vi "Multichannel Recording0.9E.vi"() -> ()   [LabVIEW 2014]
uses:
  MultiChannelScheduling 1/Enum State Typedef.ctl
  MultiChannelScheduling 1/Consumer Data_ Consumer Event Com.ctl
  MultiChannelScheduling 1/Data Producer States.ctl
  <vilib>/_DAQmxBase/Internals/DAQmxBase Read (Analog 2D DBL NChan NSamp).vi
  <vilib>/_DAQmxBase/Internals/DAQmxBase Create Channel (AI-Voltage-Basic).vi
  <vilib>/_DAQmxBase/Internals/DAQmxBase Timing (Sample Clock).vi
panel:
  out "Recording Progress (% )":dbl(slide) scale=0.0..1.0
  in  "Display Size":T1(ring)
  out "Total Iterations Needed":dbl
  out "Read Data":i32
  out "Data Producer State":T2=enum."Default"
  out "Data Consumer State":T3=enum."Default"
  in  "Open Button":bool
  in  "Tab Control":T4(tab)
  in  "Amplifier Channel 0":T5 {"Amplifier Model" items=["Select a Model", "AM 1700", "BMA 200"]}
  out "Channel 0 Graph":waveform(dbl)(graph)
  in  "User Data Channel 0":T6
  in  "Use Channel 0":bool caption="In Use?"
  out "Channel 1 Graph":waveform(dbl)(graph)
  in  "User Data Channel 1":T6
  in  "Amplifier Channel 1":T5 {"Amplifier Model" items=["Select a Model", "AM 1700", "BMA 200"]}
  in  "Use Channel 1":bool caption="In Use?"
  out "Channel 2 Graph":waveform(dbl)(graph)
  in  "User Data Channel 2":T6
  in  "Amplifier Channel 2":T5 {"Amplifier Model" items=["Select a Model", "AM 1700", "BMA 200"]}
  in  "Use Channel 2":bool caption="In Use?"
  out "Channel 3 Graph":waveform(dbl)(graph)
  in  "User Data Channel 3":T6
  in  "Amplifier Channel 3":T5 {"Amplifier Model" items=["Select a Model", "AM 1700", "BMA 200"]}
  in  "Use Channel 3":bool caption="In Use?"
  out "Overview Graph":waveform(dbl)[](graph)
  in  "Stop Preview":bool
  in  "OK Button":bool
  out "Event State":T7
  in  "Clear Display":bool
  in  "Preview Button":bool
  out "Iterations Recorded":i32
  in  "Recording Time (s)":dbl
  in  "Sample Rate":i64=1000
  in  "Stop Button":bool
  out "Start Time hr/min":string
  out "Date mm/dd/yy":string
  in  "Exit Button":bool
  in  "Record Button":bool
  # "MSU EFISH Lab Multi-Channel Electronic Pulse Recorder v0.9E (Beta 6)"
  # "Setup"
  # "Must set sample rate before you press start"
  # "Preview"
  # "Recording"
  # "Blue for On\nOrange for Off"
  # "DC"
  # "AC"
  # "Blue for AC and Orange for DC"
  # "Blue for On\nOrange for Off"
  # "DC"
  # "AC"
  # "Blue for AC and Orange for DC"
  # "Blue for On\nOrange for Off"
  # "DC"
  # "AC"
  # "Blue for AC and Orange for DC"
  # "Blue for On\nOrange for Off"
  # "DC"
  # "AC"
  # "Blue for AC and Orange for DC"
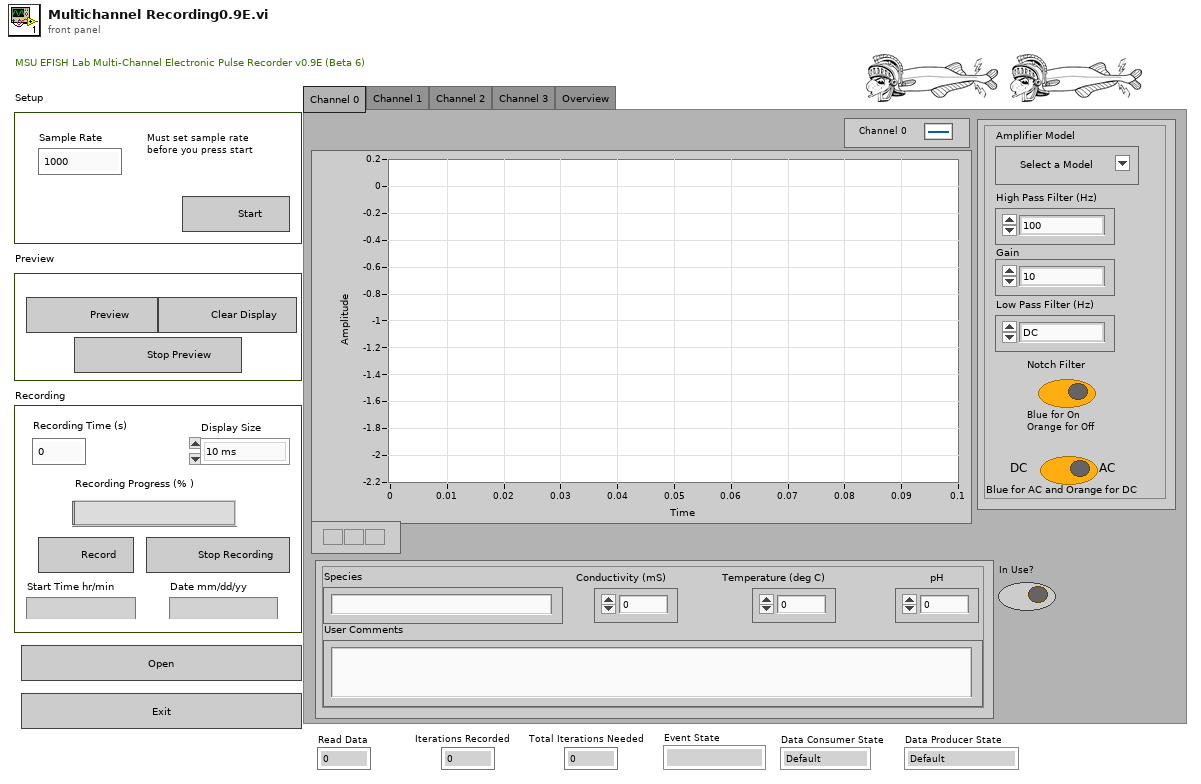
[diagram p1: front panel]
types:
  T1 = enum16{"10 ms", "100 ms", "1 Second", "10 sec", "30 sec"}
  T2 = typedef "Data Producer States.ctl" = enum16{"Read Data", "Set Sample Clock", "Default", "Exit", "Preview"}
  T3 = typedef "Consumer Data_ Consumer Event Com.ctl" = enum16{"Recording", "Create File", "Clear Memory", "Default", "End File", "Exit", "Set Sample Clock", "Preview"}
  T4 = enum32{"Channel 0", "Channel 1", "Channel 2", "Channel 3", "Overview"}
  T5 = cluster{"Low Pass Filter (Hz)":enum16{"DC", "0.1", "1", "3", "10", "30", "100", "300"}, "Gain ":enum16{"10", "20", "50", "100", "200", "500", "1000", "2k", "5k", "10k", "20k", "50k"}, "High Pass Filter (Hz)":enum16{"100", "500", "1000", "3000", "5000", "10,000", "20,000", "30,000", "50,000"}, "Notch Filter":bool, "Amplifier Model":u16, "AC/DC Switch":bool}
  T6 = cluster{"pH":dbl, "Conductivity (mS)":dbl, "Temperature (deg C)":dbl, "User Comments":string, "Species":string}
  T7 = typedef "Enum State Typedef.ctl" = enum16{"", "Open FIle", "Beginning State", "Set the Sample Clock", "Prepreview Handling", "Clear Display", "Preview Data", "Stop", "Exit", "Record", "Create File"}
  T8 = enum8{"Enabled", "Disabled", "Disabled and Grayed Out"}
  T9 = enum16{"Recording", "Create File", "Clear Memory", "Default"}
  T10 = cluster{"Refnum out":refnum<k34>, "Refnum out":refnum<k34>, "Refnum out":refnum<k34>, "Refnum out":refnum<k34>}
  T11 = cluster{"Use Channel 0":bool, "Use Channel 1":bool, "Use Channel 2":bool, "Use Channel 3":bool}
  T12 = cluster{"tdms file out":refnum<k34>, "tdms file out":refnum<k34>, "tdms file out":refnum<k34>, "tdms file out":refnum<k34>}
  T13 = cluster{"Waveform":waveform(dbl), "Waveform":waveform(dbl), "Waveform":waveform(dbl), "Waveform":waveform(dbl), waveform(dbl)[]}
  T14 = cluster{"Channel 0 Graph":refnum<vi>, "Channel 1 Graph":refnum<vi>, "Channel 2 Graph":refnum<vi>, "Channel 3 Graph":refnum<vi>, "Overview Graph":refnum<vi>}
  T15 = enum16{"Read Data", "Set Sample Clock", "Default", "Exit"}
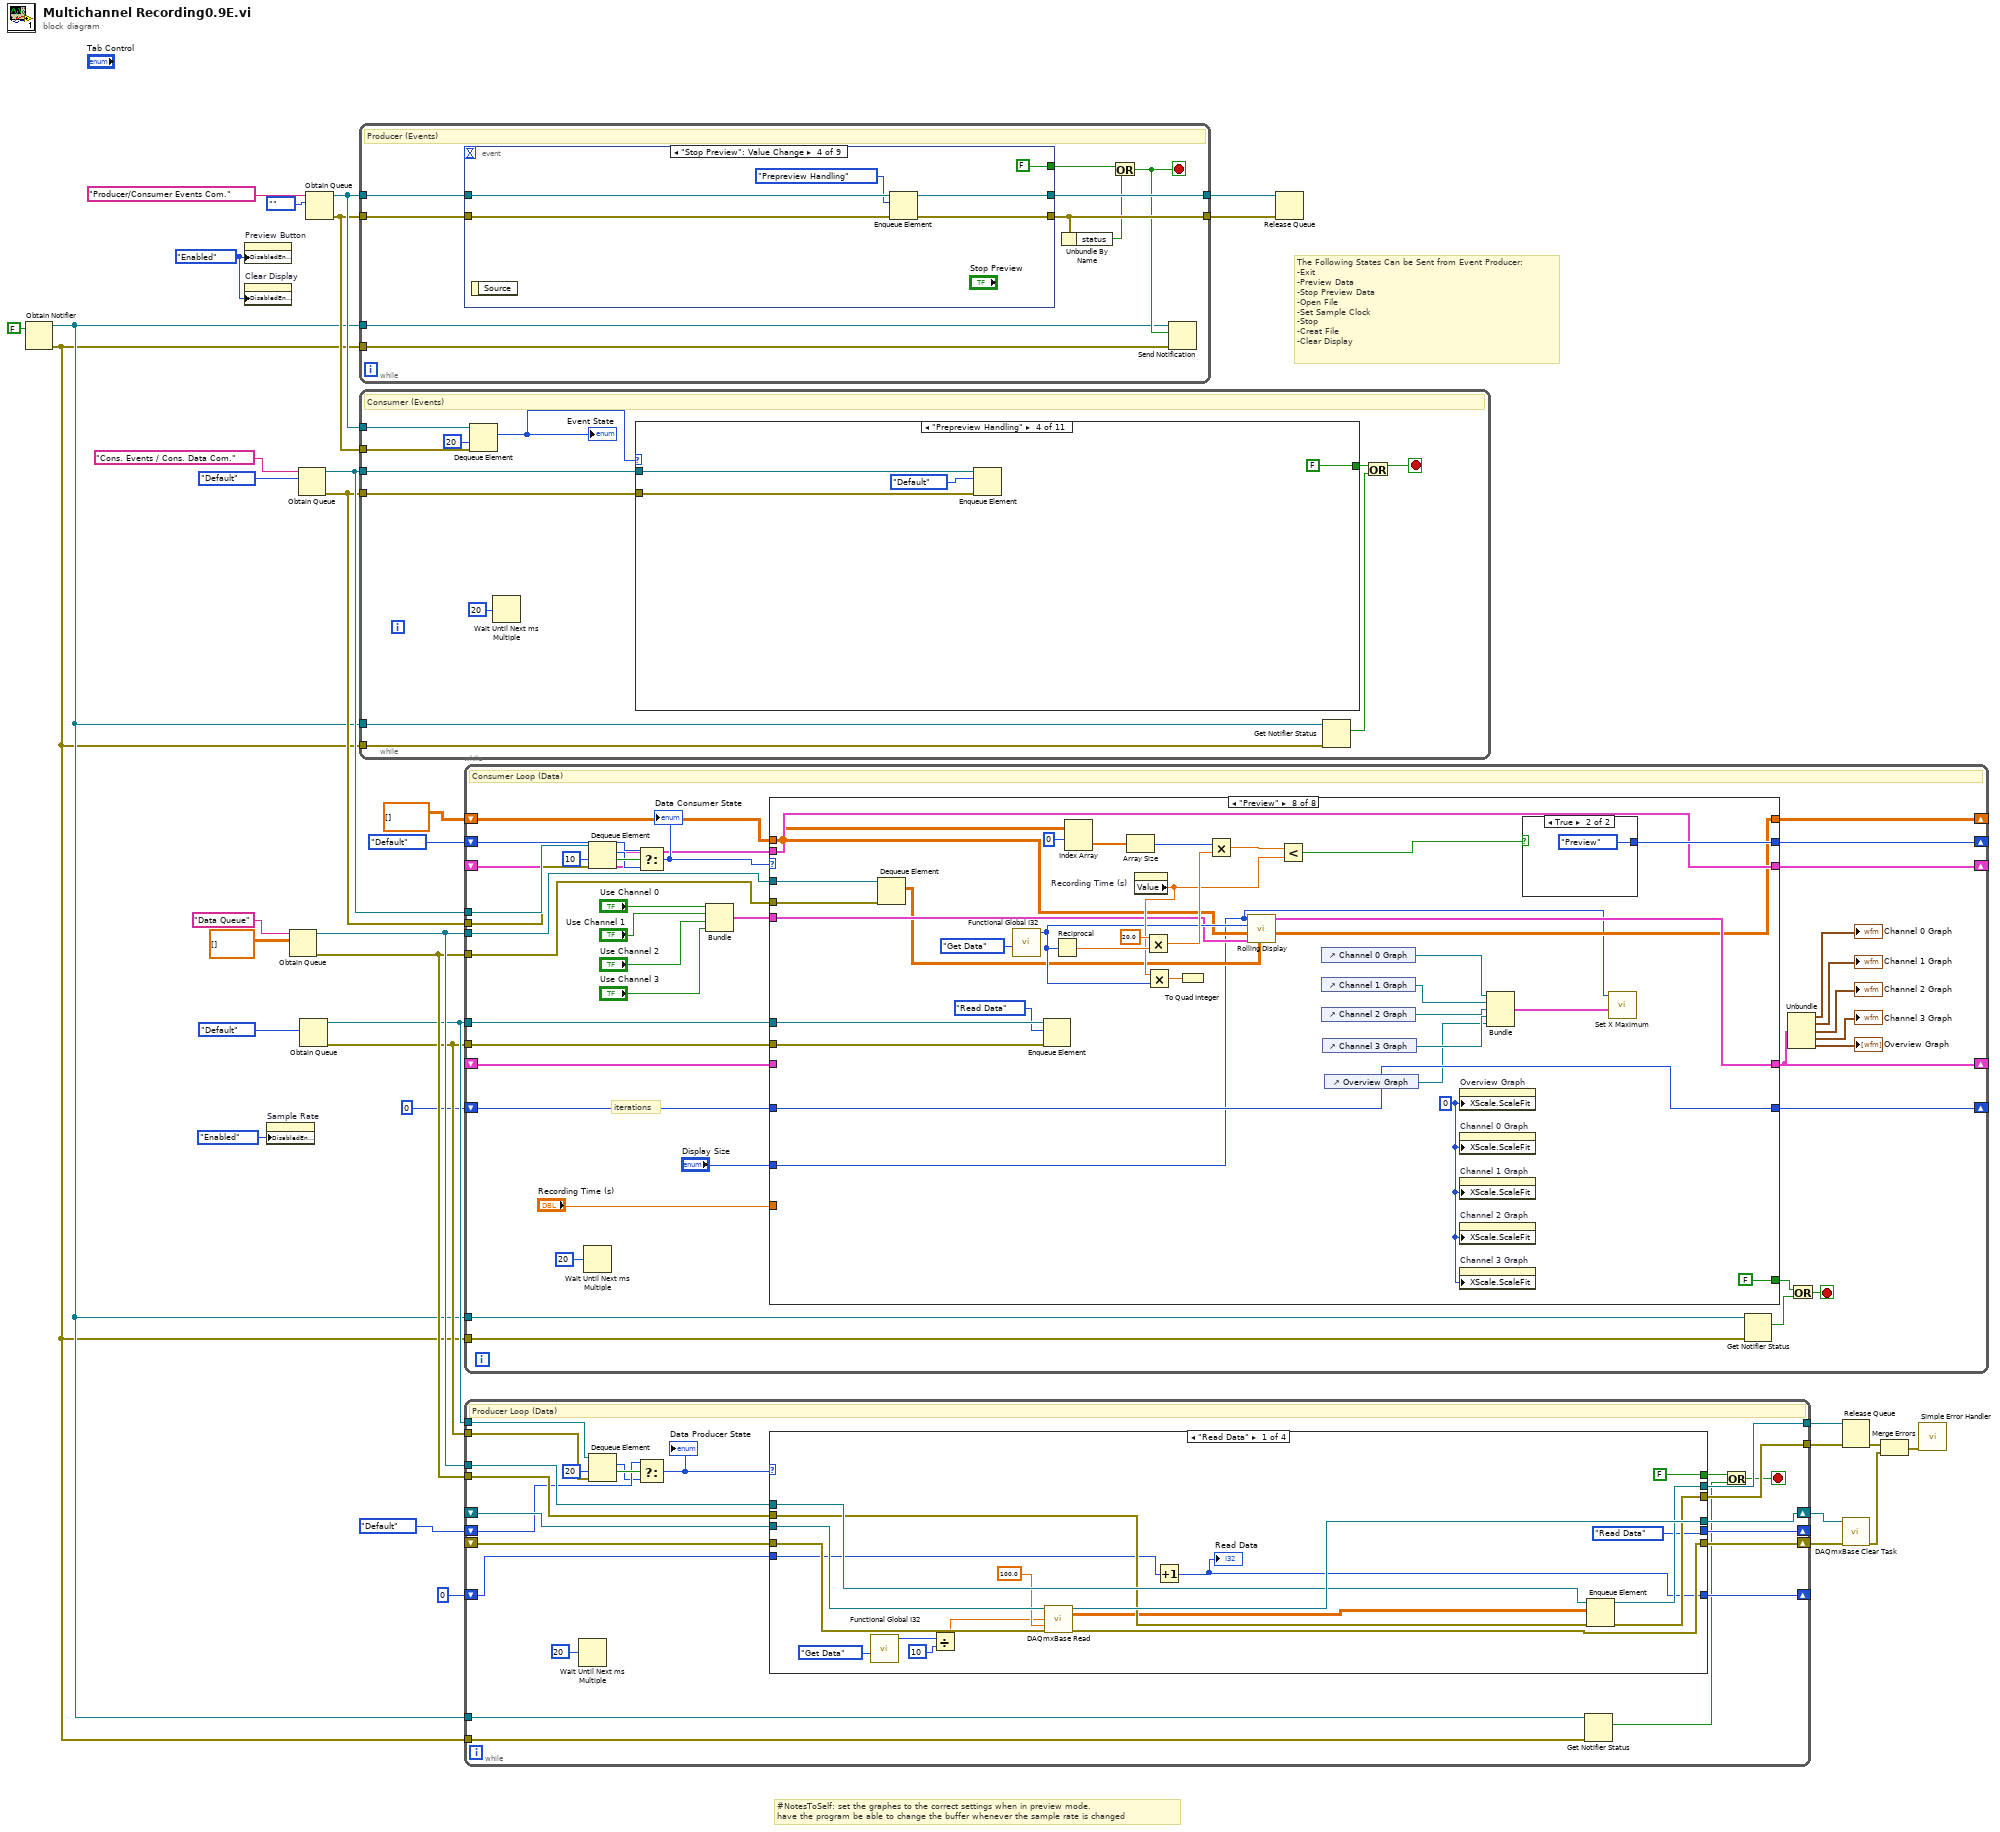
[diagram p0: block diagram]
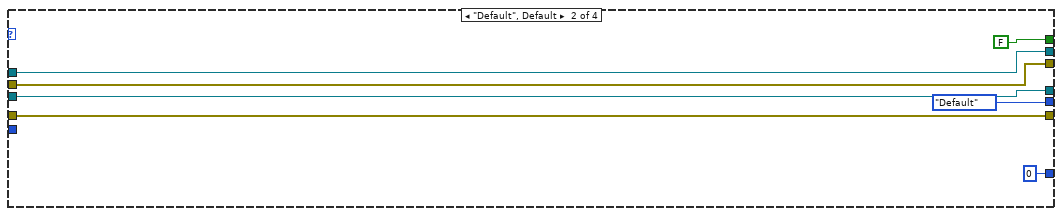
[diagram p2: hidden frame]
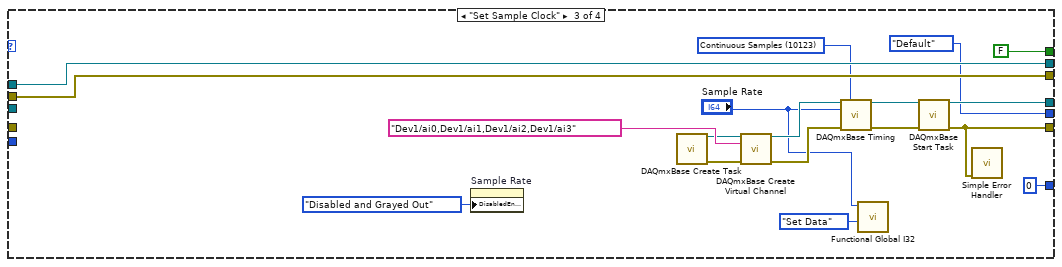
[diagram p3: hidden frame]
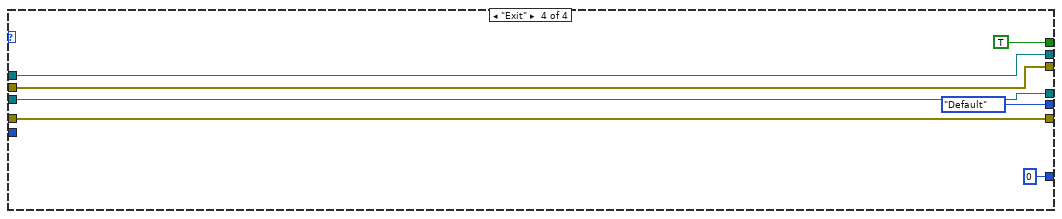
[diagram p4: hidden frame]
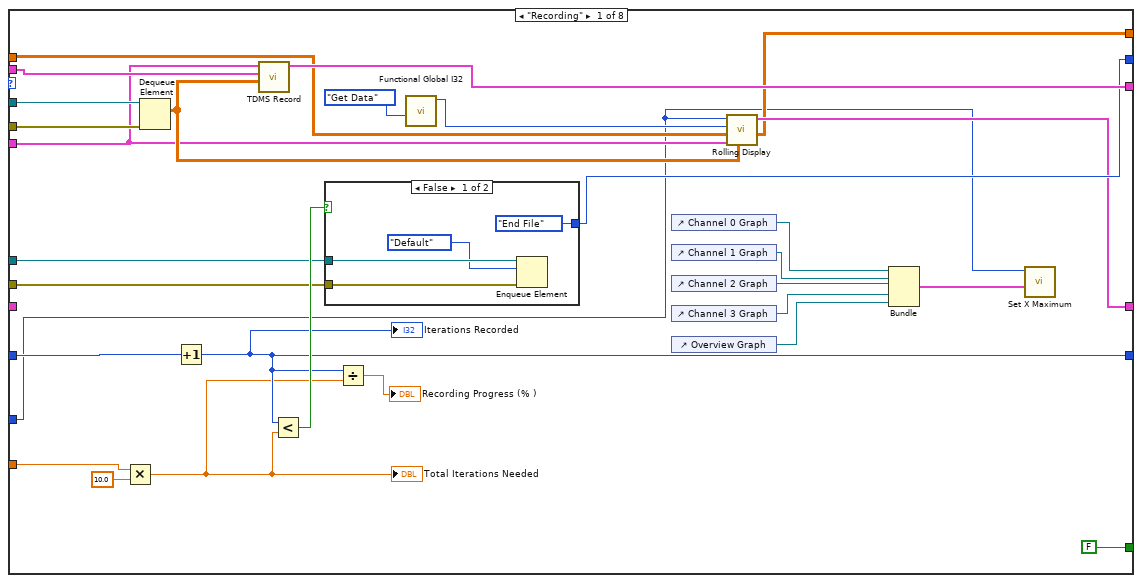
[diagram p5: hidden frame]
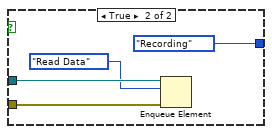
[diagram p6: hidden frame]
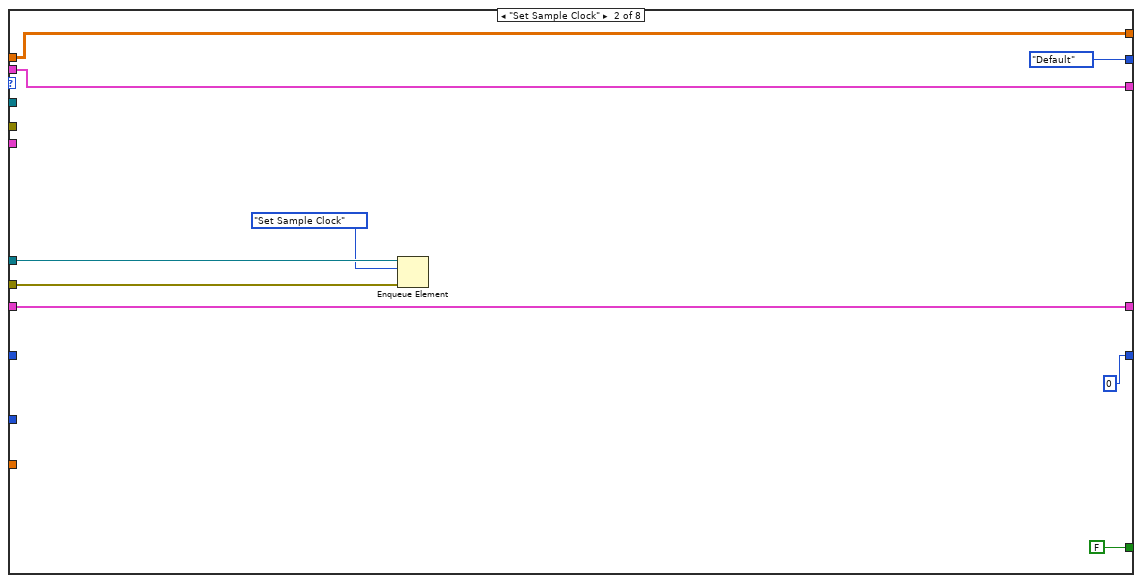
[diagram p7: hidden frame]
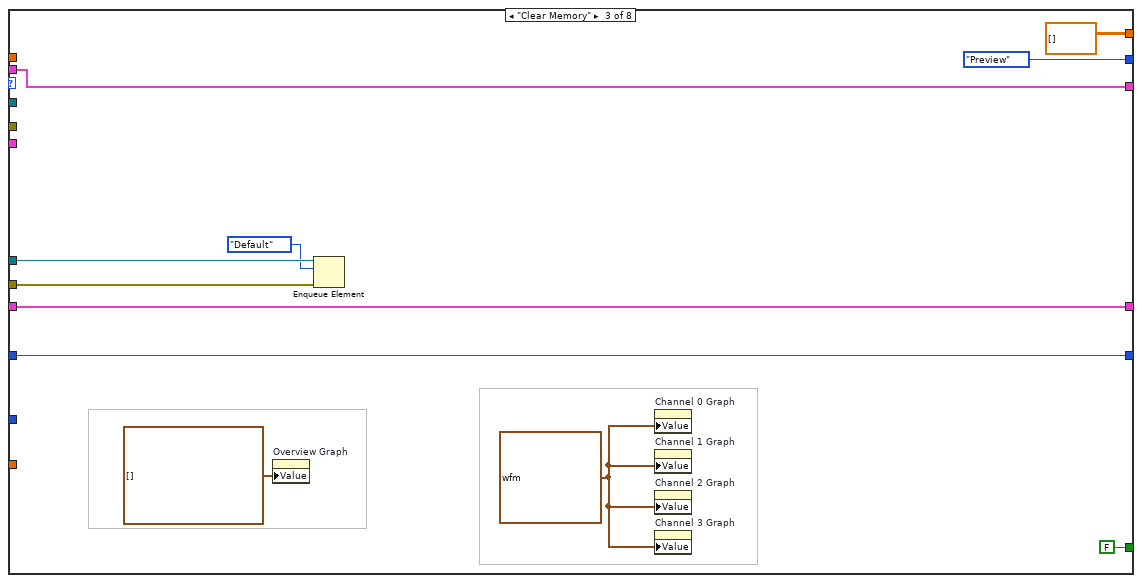
[diagram p8: hidden frame]
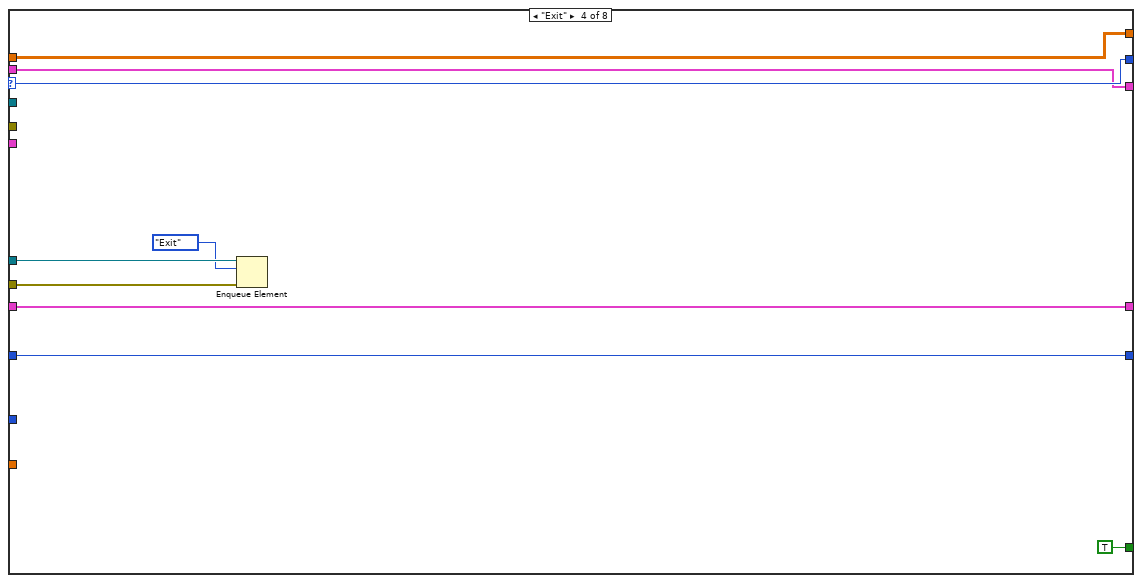
[diagram p9: hidden frame]
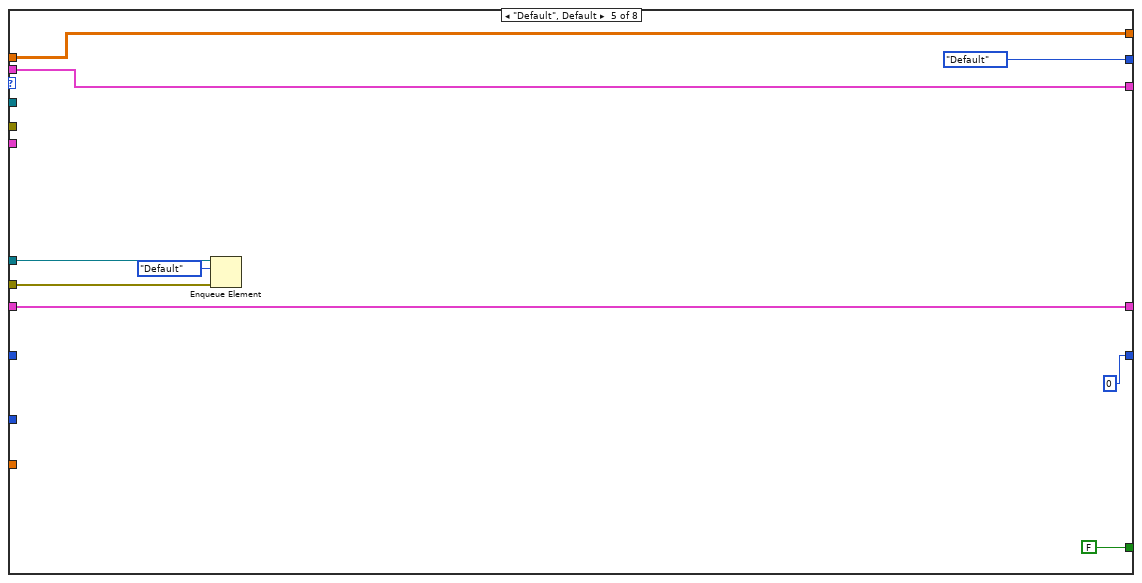
[diagram p10: hidden frame]
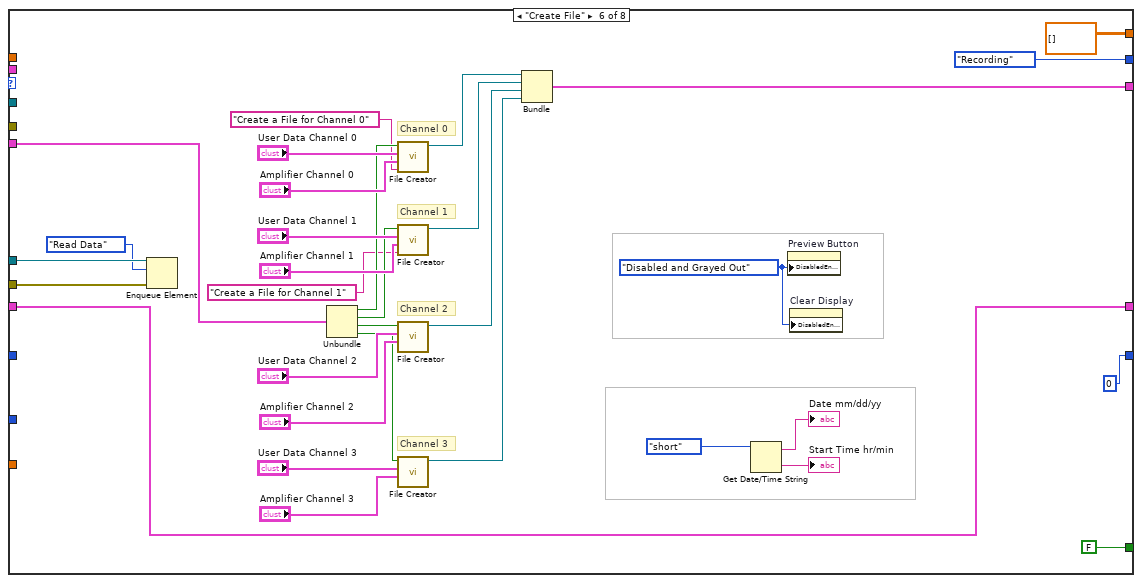
[diagram p11: hidden frame]
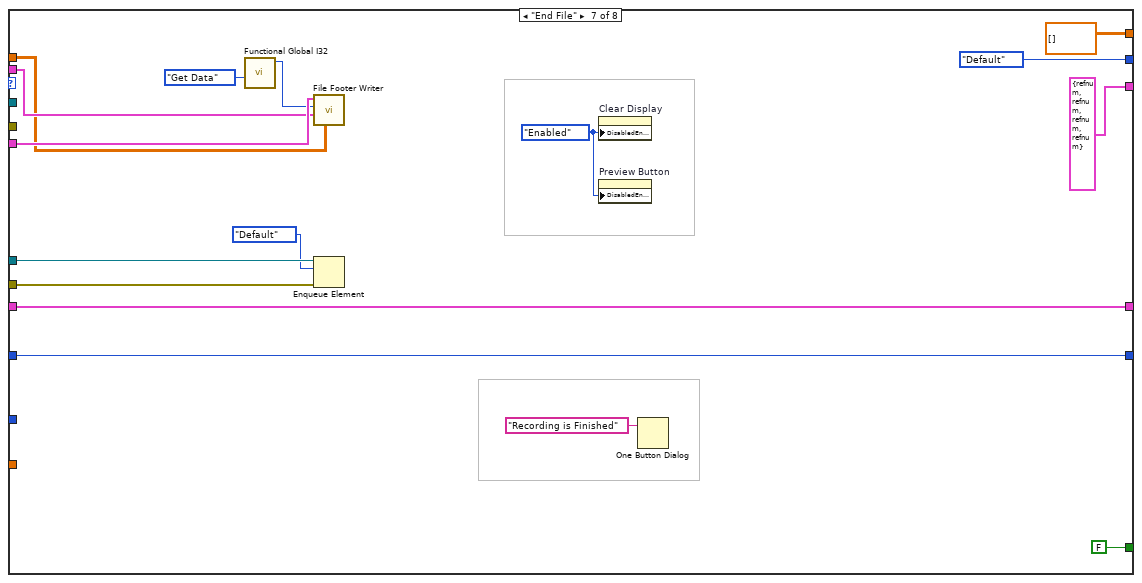
[diagram p12: hidden frame]
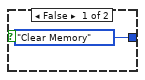
[diagram p13: hidden frame]
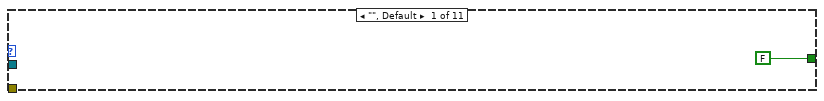
[diagram p14: hidden frame]
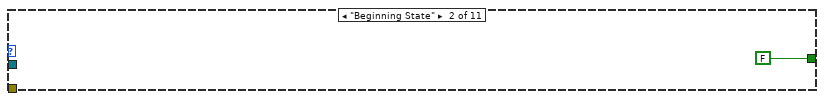
[diagram p15: hidden frame]
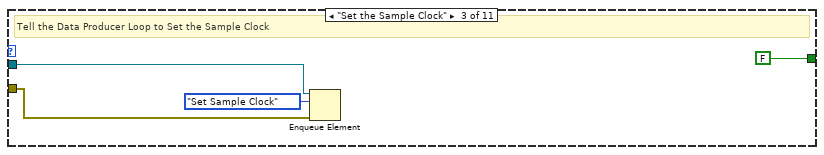
[diagram p16: hidden frame]
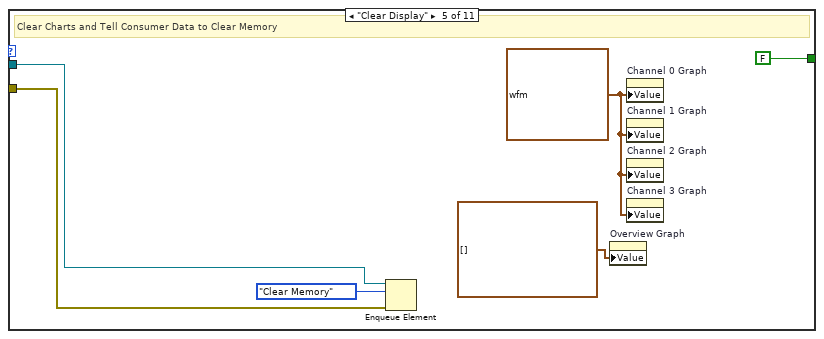
[diagram p17: hidden frame]
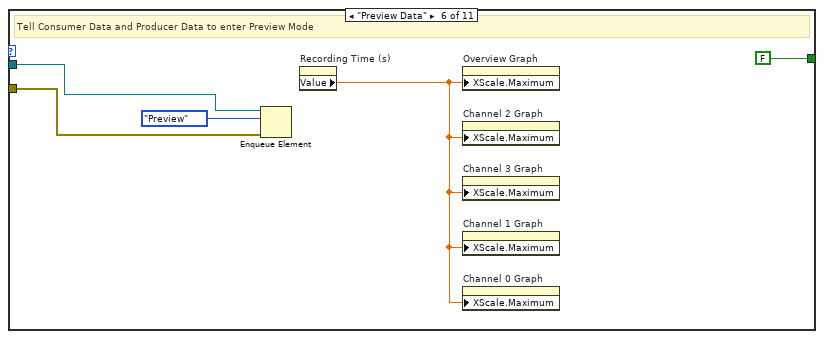
[diagram p18: hidden frame]
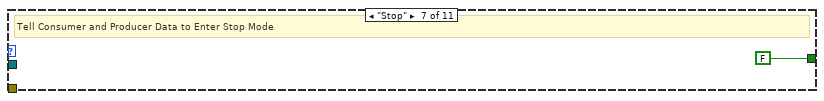
[diagram p19: hidden frame]
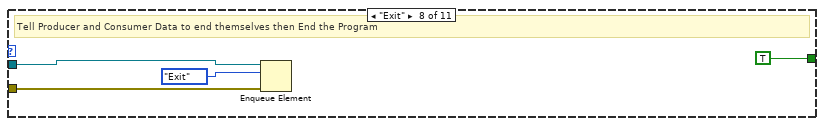
[diagram p20: hidden frame]
diagram:
  w1 = T8."Enabled" ("Disabled")
  # "#NotesToSelf: set the graphes to the correct settings when in preview mode.\nhave the program be able to change the buffer whenever the sample rate is changed"
  # "The Following States Can be Sent from Event Producer:\n-Exit\n-Preview Data\n-Stop Preview Data\n-Open File\n-Set Sample Clock\n-Stop\n-Creat File\n-Clear Display"
  n1 = Obtain Notifier(notification data type=FALSE) -> (notifier out=w3:refnum<notifier>, error out=w2:errorcluster)  [unwired: 3 in, 1 out]
  n2 = property on="Preview Button" class="Bool (strict)"("DisabledEnum"=w1) -> ()  [unwired: 2 in, 2 out]
  n3 = property on="Clear Display" class="Bool"("DisabledEnum"=w1) -> ()  [unwired: 2 in, 2 out]
  n4 = property on="Sample Rate" class="DigNum (strict)"("DisabledEnum"=T8."Enabled" ("Disabled")) -> ()  [unwired: 2 in, 2 out]
  n5 = Obtain Queue(name (unnamed)="Data Queue", element data type=dbl[][] []) -> (queue out=w29:refnum<queue>, error out=w28:errorcluster)  [unwired: 3 in, 1 out]
  n6 = Obtain Queue(name (unnamed)="Cons. Events / Cons. Data Com.", element data type=Consumer_Data__Consumer_Event_Com."Default") -> (queue out=w21:refnum<queue>, error out=w20:errorcluster)  [unwired: 3 in, 1 out]
  n7 = Obtain Queue(element data type=Data_Producer_States."Default") -> (queue out=w10:refnum<queue>, error out=w9:errorcluster)  [unwired: 4 in, 1 out]
  n8 = Obtain Queue(name (unnamed)="Producer/Consumer Events Com.", element data type=Enum_State_Typedef."" ("State")) -> (queue out=w33:refnum<queue>, error out=w32:errorcluster)  [unwired: 3 in, 1 out]
  n9 = while {
    tunnel: w33 -> [w43]
    tunnel: w32 -> [w42]
    tunnel: [w41] -> w27
    tunnel: [w40] -> w26
    tunnel: w3 -> [w36]
    tunnel: w2 -> [w35]
    stop <- w37 stop-if-true
    # "Producer (Events)"
    n10 = event shown="[3] \"Stop Preview\": Value Change" {
      selector: _ -> [_ _ _ _ _ _ _ _ _]
      dyn-events: _ -> [_ _ _ _ _ _ _ _ _]
      timeout: _ -> [_ _ _ _ _ _ _ _ _]
      tunnel: [FALSE ("Exit Button") "Exit Button" FALSE ("Exit Button") FALSE ("Exit Button") FALSE ("Exit Button") FALSE ("Exit Button") FALSE ("Exit Button") FALSE ("Exit Button") FALSE ("Exit Button")] -> w39
      tunnel: w43 -> [w45 w51 w58 w64 w70 w76 w82 w88 w94]
      tunnel: w42 -> [w44 w50 w57 w63 w69 w75 w81 w87 w93]
      tunnel: [w45 w48 w54 w60 w66 w72 w78 w84 w90] -> w41
      tunnel: [w44 w47 w53 w59 w65 w71 w77 w83 w89] -> w40
      event Timeout {
        n11 = event-data() -> ()  [unwired: 1 in, 1 out]
      }
      event "Exit Button": Value Change {
        n12 = event-data() -> ()  [unwired: 1 in, 1 out]
        n13 = Enqueue Element(queue=w51, element=Enum_State_Typedef."Exit", error in (no error)=w50) -> (queue out=w48:refnum<queue>, error out=w47:errorcluster)  [unwired: 1 in, 1 out]
      }
      event "Preview Button": Value Change {
        n14 = event-data() -> ()  [unwired: 1 in, 1 out]
        n15 = Enqueue Element(queue=w58, element=Enum_State_Typedef."Preview Data", error in (no error)=w57) -> (queue out=w54:refnum<queue>, error out=w53:errorcluster)  [unwired: 1 in, 1 out]
      }
      event "Stop Preview": Value Change {
        n16 = event-data() -> ()  [unwired: 1 in, 1 out]
        n17 = Enqueue Element(queue=w64, element=Enum_State_Typedef."Prepreview Handling", error in (no error)=w63) -> (queue out=w60:refnum<queue>, error out=w59:errorcluster)  [unwired: 1 in, 1 out]
      }
      event "Open Button": Value Change {
        n18 = event-data() -> ()  [unwired: 1 in, 1 out]
        n19 = Enqueue Element(queue=w70, element=Enum_State_Typedef."Open FIle", error in (no error)=w69) -> (queue out=w66:refnum<queue>, error out=w65:errorcluster)  [unwired: 1 in, 1 out]
      }
      event "OK Button": Value Change {
        n20 = event-data() -> ()  [unwired: 1 in, 1 out]
        n21 = Enqueue Element(queue=w76, element=Enum_State_Typedef."Set the Sample Clock", error in (no error)=w75) -> (queue out=w72:refnum<queue>, error out=w71:errorcluster)  [unwired: 1 in, 1 out]
      }
      event "Stop Button": Value Change {
        n22 = event-data() -> ()  [unwired: 1 in, 1 out]
        n23 = Enqueue Element(queue=w82, element=Enum_State_Typedef."Stop", error in (no error)=w81) -> (queue out=w78:refnum<queue>, error out=w77:errorcluster)  [unwired: 1 in, 1 out]
      }
      event "Record Button": Value Change {
        n24 = event-data() -> ()  [unwired: 1 in, 1 out]
        n25 = Enqueue Element(queue=w88, element=Enum_State_Typedef."Create File", error in (no error)=w87) -> (queue out=w84:refnum<queue>, error out=w83:errorcluster)  [unwired: 1 in, 1 out]
      }
      event "Clear Display": Value Change {
        n26 = event-data() -> ()  [unwired: 1 in, 1 out]
        n27 = Enqueue Element(queue=w94, element=Enum_State_Typedef."Clear Display", error in (no error)=w93) -> (queue out=w90:refnum<queue>, error out=w89:errorcluster)  [unwired: 1 in, 1 out]
      }
    }
    n28 = Unbundle By Name(w40) -> ("status"=w38:bool)
    n29 = Or(x=w39, y=w38) -> (x .or. y?=w37:bool)
    n30 = Send Notification(notification=w37, notifier=w36, error in (no error)=w35) -> ()  [unwired: 2 out]
  }
  n31 = while {
    tunnel: w33 -> [w106]
    tunnel: w32 -> [w105]
    tunnel: w21 -> [w104]
    tunnel: w20 -> [w103]
    tunnel: w3 -> [w98]
    tunnel: w2 -> [w97]
    stop <- w96 stop-if-true
    # "Consumer (Events)"
    n32 = Dequeue Element(queue=w106, timeout in ms (-1)=20, error in (no error)=w105) -> (element=w101:T7)  [unwired: 3 out]
    "Event State" <- w101
    n33 = Wait Until Next ms Multiple(millisecond multiple=u32 20) -> ()  [unwired: 1 out]
    n34 = case shown="\"Prepreview Handling\"" w101 {
      tunnel: w104 -> [_ _ w111 w115 w121 w125 _ w132 _ w137 _]
      tunnel: w103 -> [_ _ w110 w114 w120 w124 _ w131 _ w136 _]
      tunnel: [FALSE FALSE FALSE FALSE FALSE FALSE FALSE TRUE FALSE FALSE FALSE] -> w102
      frame "", Default {
      }
      frame "Beginning State" {
      }
      frame "Set the Sample Clock" {
        # "Tell the Data Producer Loop to Set the Sample Clock"
        n35 = Enqueue Element(queue=w111, element=Consumer_Data__Consumer_Event_Com."Set Sample Clock", error in (no error)=w110) -> ()  [unwired: 1 in, 3 out]
      }
      frame "Prepreview Handling" {
        n36 = Enqueue Element(queue=w115, element=Consumer_Data__Consumer_Event_Com."Default", error in (no error)=w114) -> ()  [unwired: 1 in, 3 out]
      }
      frame "Clear Display" {
        w118 = waveform(dbl) {"t0"=timestamp(0 s since 1904-01-01), "dt"=1.0, "Y"=[]} ("Channel 0 Graph")
        # "Clear Charts and Tell Consumer Data to Clear Memory"
        n37 = Enqueue Element(queue=w121, element=Consumer_Data__Consumer_Event_Com."Clear Memory", error in (no error)=w120) -> ()  [unwired: 1 in, 3 out]
        n38 = property on="Overview Graph" class="WFGraph (strict)"("Value"=waveform(dbl)[] [] ("Overview Graph")) -> ()  [unwired: 2 in, 2 out]
        n39 = property on="Channel 0 Graph" class="WFGraph (strict)"("Value"=w118) -> ()  [unwired: 2 in, 2 out]
        n40 = property on="Channel 1 Graph" class="WFGraph (strict)"("Value"=w118) -> ()  [unwired: 2 in, 2 out]
        n41 = property on="Channel 2 Graph" class="WFGraph (strict)"("Value"=w118) -> ()  [unwired: 2 in, 2 out]
        n42 = property on="Channel 3 Graph" class="WFGraph (strict)"("Value"=w118) -> ()  [unwired: 2 in, 2 out]
      }
      frame "Preview Data" {
        # "Tell Consumer Data and Producer Data to enter Preview Mode"
        n43 = Enqueue Element(queue=w125, element=Consumer_Data__Consumer_Event_Com."Preview", error in (no error)=w124) -> ()  [unwired: 1 in, 3 out]
        n44 = property on="Recording Time (s)" class="DigNum (strict)"() -> ("Value"=w126:dbl)  [unwired: 2 in, 2 out]
        n45 = property on="Overview Graph" class="WFGraph (strict)"("XScale.Maximum"=w126) -> ()  [unwired: 2 in, 2 out]
        n46 = property on="Channel 2 Graph" class="WFGraph (strict)"("XScale.Maximum"=w126) -> ()  [unwired: 2 in, 2 out]
        n47 = property on="Channel 3 Graph" class="WFGraph (strict)"("XScale.Maximum"=w126) -> ()  [unwired: 2 in, 2 out]
        n48 = property on="Channel 1 Graph" class="WFGraph (strict)"("XScale.Maximum"=w126) -> ()  [unwired: 2 in, 2 out]
        n49 = property on="Channel 0 Graph" class="WFGraph (strict)"("XScale.Maximum"=w126) -> ()  [unwired: 2 in, 2 out]
      }
      frame "Stop" {
        # "Tell Consumer and Producer Data to Enter Stop Mode"
      }
      frame "Exit" {
        # "Tell Producer and Consumer Data to end themselves then End the Program"
        n50 = Enqueue Element(queue=w132, element=Consumer_Data__Consumer_Event_Com."Exit", error in (no error)=w131) -> ()  [unwired: 1 in, 3 out]
      }
      frame "Record" {
        # "(I dont think that this case will exist)"
      }
      frame "Create File" {
        w134 = u8 0 ("X Scale.Scale Fit")
        # "Let Consumer Data Create File"
        n51 = Enqueue Element(queue=w137, element=Consumer_Data__Consumer_Event_Com."Create File", error in (no error)=w136) -> ()  [unwired: 1 in, 3 out]
        n52 = property on="Overview Graph" class="WFGraph (strict)"("XScale.ScaleFit"=w134) -> ()  [unwired: 2 in, 2 out]
        n53 = property on="Channel 3 Graph" class="WFGraph (strict)"("XScale.ScaleFit"=w134) -> ()  [unwired: 2 in, 2 out]
        n54 = property on="Channel 2 Graph" class="WFGraph (strict)"("XScale.ScaleFit"=w134) -> ()  [unwired: 2 in, 2 out]
        n55 = property on="Channel 1 Graph" class="WFGraph (strict)"("XScale.ScaleFit"=w134) -> ()  [unwired: 2 in, 2 out]
        n56 = property on="Channel 0 Graph" class="WFGraph (strict)"("XScale.ScaleFit"=w134) -> ()  [unwired: 2 in, 2 out]
      }
      frame "Open FIle" {
        # "Tell the Data Consumer to Create the File"
        n57 = call "File Dialog"() -> ("selected path"=w139:path)  [unwired: 12 in, 3 out]
        n58 = call <vilib>:"TDMS - File Viewer.vi"("file path"=w139) -> ()  [unwired: 5 in, 2 out]
      }
    }
    n59 = Get Notifier Status(notifier=w98, error in (no error)=w97) -> (current notification=w95:bool)  [unwired: 4 out]
    n60 = Or(x=w102, y=w95) -> (x .or. y?=w96:bool)
  }
  n61 = while {
    tunnel: w29 -> [w171]
    tunnel: w28 -> [w170]
    tunnel: w21 -> [w178]
    tunnel: w20 -> [w177]
    shift-right: [w172] -> _
    shift-left: Consumer_Data__Consumer_Event_Com."Default" -> [w173]
    shift-right: [w166] -> _
    shift-left: dbl[][] [] -> [w169]
    shift-right: [w165] -> _
    shift-left: _ -> [w164]
    tunnel: w10 -> [w162]
    tunnel: w9 -> [w161]
    shift-right: [w157] -> _
    shift-left: 0 -> [w159]
    tunnel: w3 -> [w151]
    tunnel: w2 -> [w150]
    shift-right: [w143] -> _
    shift-left: _ -> [w142]
    stop <- w153 stop-if-true
    # "iterations"
    # "Consumer Loop (Data)"
    n62 = Wait Until Next ms Multiple(millisecond multiple=u32 20) -> ()  [unwired: 1 out]
    n63 = Dequeue Element(queue=w178, timeout in ms (-1)=10, error in (no error)=w177) -> (element=w175:T3, timed out?=w176:bool)  [unwired: 2 out]
    n64 = Select(t=w173, s=w176, f=w175) -> (s? t:f=w174:T3)
    "Data Consumer State" <- w174
    n65 = Bundle("Use Channel 0"="Use Channel 0", "Use Channel 1"="Use Channel 1", "Use Channel 2"="Use Channel 2", "Use Channel 3"="Use Channel 3") -> (w167:T11)  [unwired: 1 in]
    n66 = case shown="\"Preview\"" w174 {
      selector: w174 -> [_ _ _ w242 _ _ _ _]
      tunnel: [w199 Consumer_Data__Consumer_Event_Com."Default" Consumer_Data__Consumer_Event_Com."Preview" w242 T9."Default" Consumer_Data__Consumer_Event_Com."Recording" Consumer_Data__Consumer_Event_Com."Default" w325] -> w172
      tunnel: w171 -> [w206 _ _ _ _ _ _ w335]
      tunnel: w170 -> [w205 _ _ _ _ _ _ w334]
      tunnel: [FALSE FALSE FALSE TRUE FALSE FALSE FALSE FALSE] -> w152
      tunnel: w169 -> [w192 w221 _ w243 w251 _ w299 w313]
      tunnel: w167 -> [w191 _ _ _ _ w279 w301 w312]
      tunnel: [w189 w221 dbl[][] [] ("Output Decimated Data") w243 w251 dbl[][] [] ("Output Decimated Data") dbl[][] [] ("Output Data") w309] -> w166
      tunnel: [w204 w220 w232 w241 w250 w262 T10 {"Refnum out"=refnum, "Refnum out"=refnum, "Refnum out"=refnum, "Refnum out"=refnum} ("Output TDMS File Cluster") w315] -> w165
      tunnel: w164 -> [w196 w220 w232 w241 w250 _ w300 w315]
      tunnel: w162 -> [w198 w224 w231 w240 w248 w261 w294 w323]
      tunnel: w161 -> [w197 w223 w230 w239 w247 w260 w293 w322]
      tunnel: w159 -> [w203 _ w228 w237 _ _ w291 w320]
      tunnel: "Recording Time (s)" -> [w202 _ _ _ _ _ _ _]
      tunnel: [w182 0 w228 w237 0 0 w291 w320] -> w157
      tunnel: [w190 w216 w227 w236 w245 w255 w289 w310] -> w143
      tunnel: w142 -> [_ w216 w227 w236 w245 w255 w289 _]
      tunnel: "Display Size" -> [w179 _ _ _ _ _ _ w302]
      frame "Recording" {
        n67 = Multiply(x=w202, y=10.0) -> (x*y=w181:dbl)
        "Total Iterations Needed" <- w181
        n68 = Dequeue Element(queue=w206, error in (no error)=w205) -> (element=w193:dbl[][])  [unwired: 1 in, 3 out]
        n69 = Increment(x=w203) -> (x+1=w182:i32)
        "Iterations Recorded" <- w182
        n70 = call "TDMS Record.vi"("Data"=w193, "Input TDMS File Cluster"=w196, "In Use Cluster"=w191) -> ("Output TDMS File Cluster"=w204:T12)  [unwired: 7 in, 1 out]
        n71 = Less?(x=w182, y=w181) -> (x < y?=w200:bool)
        n72 = case shown="False" w200 {
          tunnel: [Consumer_Data__Consumer_Event_Com."End File" Consumer_Data__Consumer_Event_Com."Recording"] -> w199
          tunnel: w198 -> [w210 w214]
          tunnel: w197 -> [w209 w213]
          frame False {
            n73 = Enqueue Element(queue=w210, element=Data_Producer_States."Default", error in (no error)=w209) -> ()  [unwired: 1 in, 3 out]
          }
          frame True {
            n74 = Enqueue Element(queue=w214, element=Data_Producer_States."Read Data", error in (no error)=w213) -> ()  [unwired: 1 in, 3 out]
          }
        }
        n75 = Divide(x=w182, y=w181) -> (x/y=→"Recording Progress (% )":dbl)
        n76 = call "Functional Global I32.vi"("Enum"=enum16{"Set Data", "Get Data"}."Get Data") -> ("Integer"=w194:i32)  [unwired: 10 in]
        n77 = control-ref of="Channel 0 Graph"() -> (w188:refnum<vi>)
        n78 = control-ref of="Channel 1 Graph"() -> (w187:refnum<vi>)
        n79 = control-ref of="Channel 2 Graph"() -> (w186:refnum<vi>)
        n80 = control-ref of="Channel 3 Graph"() -> (w185:refnum<vi>)
        n81 = control-ref of="Overview Graph"() -> (w184:refnum<vi>)
        n82 = call "Rolling Display.vi"("Input Data"=w193, "Channels in Use"=w191, "Old Data"=w192, "Sample Rate"=w194, "Display Size"=w179) -> ("Output Array Values"=w189:dbl[][], "Output Waveform Cluster"=w190:T13)  [unwired: 5 in]
        n83 = Bundle("Channel 0 Graph"=w188, "Channel 1 Graph"=w187, "Channel 2 Graph"=w186, "Channel 3 Graph"=w185, "Overview Graph"=w184) -> (w183:T14)  [unwired: 1 in]
        n84 = call "Set X Maximum.vi"("output cluster"=w183, "Display Size"=w179) -> ()  [unwired: 10 in]
      }
      frame "Set Sample Clock" {
        n85 = Enqueue Element(queue=w224, element=Data_Producer_States."Set Sample Clock", error in (no error)=w223) -> ()  [unwired: 1 in, 3 out]
      }
      frame "Clear Memory" {
        w226 = waveform(dbl) {"t0"=timestamp(0 s since 1904-01-01), "dt"=1.0, "Y"=[]} ("Channel 0 Graph")
        n86 = property on="Overview Graph" class="WFGraph (strict)"("Value"=waveform(dbl)[] [] ("Overview Graph")) -> ()  [unwired: 2 in, 2 out]
        n87 = Enqueue Element(queue=w231, element=Data_Producer_States."Default", error in (no error)=w230) -> ()  [unwired: 1 in, 3 out]
        n88 = property on="Channel 0 Graph" class="WFGraph (strict)"("Value"=w226) -> ()  [unwired: 2 in, 2 out]
        n89 = property on="Channel 1 Graph" class="WFGraph (strict)"("Value"=w226) -> ()  [unwired: 2 in, 2 out]
        n90 = property on="Channel 2 Graph" class="WFGraph (strict)"("Value"=w226) -> ()  [unwired: 2 in, 2 out]
        n91 = property on="Channel 3 Graph" class="WFGraph (strict)"("Value"=w226) -> ()  [unwired: 2 in, 2 out]
      }
      frame "Exit" {
        n92 = Enqueue Element(queue=w240, element=Data_Producer_States."Exit", error in (no error)=w239) -> ()  [unwired: 1 in, 3 out]
      }
      frame "Default", Default {
        n93 = Enqueue Element(queue=w248, element=Data_Producer_States."Default", error in (no error)=w247) -> ()  [unwired: 1 in, 3 out]
      }
      frame "Create File" {
        w254 = T8."Disabled and Grayed Out" ("Disabled")
        # "Channel 3"
        # "Channel 2"
        # "Channel 1"
        # "Channel 0"
        n94 = Enqueue Element(queue=w261, element=Data_Producer_States."Read Data", error in (no error)=w260) -> ()  [unwired: 1 in, 3 out]
        n95 = Unbundle(w279) -> ("Use Channel 0"=w272:bool, "Use Channel 1"=w271:bool, "Use Channel 2"=w270:bool, "Use Channel 3"=w269:bool)
        n96 = call "File Creator.vi"("prompt"="Create a File for Channel 0", "Amplifier Channel 1"="Amplifier Channel 0", "User Data Channel 1"="User Data Channel 0", "Use Channel in"=w272) -> ("Refnum out"=w268:refnum<k34>)  [unwired: 6 in, 1 out]
        n97 = call "File Creator.vi"("prompt"="Create a File for Channel 1", "Amplifier Channel 1"="Amplifier Channel 1", "User Data Channel 1"="User Data Channel 1", "Use Channel in"=w271) -> ("Refnum out"=w267:refnum<k34>)  [unwired: 6 in, 1 out]
        n98 = call "File Creator.vi"("Amplifier Channel 1"="Amplifier Channel 2", "User Data Channel 1"="User Data Channel 2", "Use Channel in"=w270) -> ("Refnum out"=w266:refnum<k34>)  [unwired: 7 in, 1 out]
        n99 = call "File Creator.vi"("Amplifier Channel 1"="Amplifier Channel 3", "User Data Channel 1"="User Data Channel 3", "Use Channel in"=w269) -> ("Refnum out"=w265:refnum<k34>)  [unwired: 7 in, 1 out]
        n100 = Bundle("Refnum out"=w268, "Refnum out"=w267, "Refnum out"=w266, "Refnum out"=w265) -> (w262:T10)  [unwired: 1 in]
        n101 = Get Date/Time String(date format (0)=enum16{"short", "long", "abbreviated"}."short") -> (date string=→"Date mm/dd/yy":string, time string=→"Start Time hr/min":string)  [unwired: 2 in]
        n102 = property on="Preview Button" class="Bool (strict)"("DisabledEnum"=w254) -> ()  [unwired: 2 in, 2 out]
        n103 = property on="Clear Display" class="Bool"("DisabledEnum"=w254) -> ()  [unwired: 2 in, 2 out]
      }
      frame "End File" {
        w288 = T8."Enabled" ("Disabled")
        n104 = call "Functional Global I32.vi"("Enum"=enum16{"Set Data", "Get Data"}."Get Data") -> ("Integer"=w286:i32)  [unwired: 10 in]
        n105 = call "File Footer Writer.vi"("Old Data"=w299, "TDMS File Cluster"=w300, "Sample Rate"=w286, "In Use Cluster"=w301) -> ()  [unwired: 7 in, 1 out]
        n106 = Enqueue Element(queue=w294, element=Data_Producer_States."Default", error in (no error)=w293) -> ()  [unwired: 1 in, 3 out]
        n107 = property on="Clear Display" class="Bool"("DisabledEnum"=w288) -> ()  [unwired: 2 in, 2 out]
        n108 = property on="Preview Button" class="Bool (strict)"("DisabledEnum"=w288) -> ()  [unwired: 2 in, 2 out]
        n109 = One Button Dialog(message="Recording is Finished") -> ()  [unwired: 1 in, 1 out]
      }
      frame "Preview" {
        w318 = u8 0 ("X Scale.Scale Fit")
        n110 = Dequeue Element(queue=w335, error in (no error)=w334) -> (element=w311:dbl[][])  [unwired: 1 in, 3 out]
        n111 = call "Functional Global I32.vi"("Enum"=enum16{"Set Data", "Get Data"}."Get Data") -> ("Integer"=w314:i32)  [unwired: 10 in]
        n112 = Enqueue Element(queue=w323, element=Data_Producer_States."Read Data", error in (no error)=w322) -> ()  [unwired: 1 in, 3 out]
        n113 = Reciprocal(x=w314) -> (1/x=w333:dbl)
        n114 = Index Array(array=w313, index (row)=0) -> (element=w329:dbl[])  [unwired: 1 in]
        n115 = Array Size(array=w329) -> (size(s)=w328:i32)
        n116 = property on="Recording Time (s)" class="DigNum (strict)"() -> ("Value"=w317:dbl)  [unwired: 2 in, 2 out]
        n117 = Multiply(x=20.0, y=w333) -> (x*y=w331:dbl)
        n118 = Multiply(x=w317, y=w314) -> (x*y=w316:dbl)
        n119 = To Quad Integer(1:w316) -> ()  [unwired: 1 out]
        n120 = Multiply(x=w328, y=w331) -> (x*y=w327:dbl)
        n121 = call "Rolling Display.vi"("Input Data"=w311, "Channels in Use"=w312, "Old Data"=w313, "Sample Rate"=w314, "Display Size"=w302) -> ("Output Array Values"=w309:dbl[][], "Output Waveform Cluster"=w310:T13)  [unwired: 5 in]
        n122 = Less?(x=w327, y=w317) -> (x < y?=w326:bool)
        n123 = control-ref of="Channel 0 Graph"() -> (w307:refnum<vi>)
        n124 = control-ref of="Channel 1 Graph"() -> (w306:refnum<vi>)
        n125 = control-ref of="Channel 2 Graph"() -> (w305:refnum<vi>)
        n126 = control-ref of="Channel 3 Graph"() -> (w304:refnum<vi>)
        n127 = control-ref of="Overview Graph"() -> (w303:refnum<vi>)
        n128 = property on="Overview Graph" class="WFGraph (strict)"("XScale.ScaleFit"=w318) -> ()  [unwired: 2 in, 2 out]
        n129 = property on="Channel 0 Graph" class="WFGraph (strict)"("XScale.ScaleFit"=w318) -> ()  [unwired: 2 in, 2 out]
        n130 = property on="Channel 1 Graph" class="WFGraph (strict)"("XScale.ScaleFit"=w318) -> ()  [unwired: 2 in, 2 out]
        n131 = property on="Channel 2 Graph" class="WFGraph (strict)"("XScale.ScaleFit"=w318) -> ()  [unwired: 2 in, 2 out]
        n132 = property on="Channel 3 Graph" class="WFGraph (strict)"("XScale.ScaleFit"=w318) -> ()  [unwired: 2 in, 2 out]
        n133 = Bundle("Channel 0 Graph"=w307, "Channel 1 Graph"=w306, "Channel 2 Graph"=w305, "Channel 3 Graph"=w304, "Overview Graph"=w303) -> (w308:T14)  [unwired: 1 in]
        n134 = case shown="True" w326 {
          tunnel: [Consumer_Data__Consumer_Event_Com."Clear Memory" Consumer_Data__Consumer_Event_Com."Preview"] -> w325
          frame False {
          }
          frame True {
          }
        }
        n135 = call "Set X Maximum.vi"("output cluster"=w308, "Display Size"=w302) -> ()  [unwired: 10 in]
      }
    }
    n136 = Get Notifier Status(notifier=w151, error in (no error)=w150) -> (current notification=w149:bool)  [unwired: 4 out]
    n137 = Unbundle(w143) -> ("Waveform"=→"Channel 0 Graph":waveform(dbl), "Waveform"=→"Channel 1 Graph":waveform(dbl), "Waveform"=→"Channel 2 Graph":waveform(dbl), "Waveform"=→"Channel 3 Graph":waveform(dbl), →"Overview Graph":waveform(dbl)[])
    n138 = Or(x=w152, y=w149) -> (x .or. y?=w153:bool)
  }
  n139 = while {
    tunnel: w29 -> [w361]
    tunnel: w28 -> [w358]
    tunnel: [w360] -> w25
    tunnel: [w359] -> w24
    shift-right: [w346] -> _
    shift-left: Data_Producer_States."Default" -> [w339]
    shift-right: [w357] -> w18
    shift-left: _ -> [w355]
    shift-right: [w356] -> w17
    shift-left: _ -> [w354]
    tunnel: w10 -> [w351]
    tunnel: w9 -> [w350]
    shift-right: [w344] -> _
    shift-left: 0 -> [w345]
    tunnel: w3 -> [w341]
    tunnel: w2 -> [w340]
    stop <- w343 stop-if-true
    # "Producer Loop (Data)"
    n140 = Wait Until Next ms Multiple(millisecond multiple=u32 20) -> ()  [unwired: 1 out]
    n141 = Dequeue Element(queue=w351, timeout in ms (-1)=20, error in (no error)=w350) -> (element=w338:T2, timed out?=w349:bool)  [unwired: 2 out]
    n142 = Select(t=w339, s=w349, f=w338) -> (s? t:f=w348:T2)
    "Data Producer State" <- w348
    n143 = case shown="\"Read Data\"" w348 {
      tunnel: w361 -> [w375 w386 w396 w407]
      tunnel: [w373 w386 w396 w407] -> w360
      tunnel: [w372 w385 w395 w408] -> w359
      tunnel: w358 -> [w374 w385 w395 w408]
      tunnel: [w377 w384 w397 w409] -> w357
      tunnel: [w376 w383 w387 w410] -> w356
      tunnel: w355 -> [w379 w384 _ w409]
      tunnel: w354 -> [w378 w383 _ w410]
      tunnel: [FALSE FALSE FALSE TRUE] -> w352
      tunnel: [Data_Producer_States."Read Data" Data_Producer_States."Default" T15."Default" Data_Producer_States."Default"] -> w346
      tunnel: w345 -> [w368 _ _ _]
      tunnel: [w367 0 0 0] -> w344
      frame "Read Data" {
        n144 = call "Functional Global I32.vi"("Enum"=enum16{"Set Data", "Get Data"}."Get Data") -> ("Integer"=w364:i32)  [unwired: 10 in]
        n145 = Divide(x=w364, y=10) -> (x/y=w363:dbl)
        n146 = call-poly <vilib>:"DAQmxBase Read.vi"("task/channels in"=w379, "number of samples per channel"=w363, "timeout"=100.0, "error in"=w378) -> ("task out"=w377:refnum<k21>, "data"=w362:dbl[][], "error out"=w376:errorcluster)  [unwired: 9 in]
        n147 = Increment(x=w368) -> (x+1=w367:i32)
        "Read Data" <- w367
        n148 = Enqueue Element(queue=w375, element=w362, error in (no error)=w374) -> (queue out=w373:refnum<queue>, error out=w372:errorcluster)  [unwired: 1 in, 1 out]
      }
      frame "Default", Default {
      }
      frame "Set Sample Clock" {
        w388 = 10123 items=["Finite Samples"=10178, "Continuous Samples"=10123, "Hardware Timed Single Point"=12522] ("sample mode")
        n149 = property on="Sample Rate" class="DigNum (strict)"("DisabledEnum"=T8."Disabled and Grayed Out" ("Disabled")) -> ()  [unwired: 2 in, 2 out]
        n150 = call <vilib>:"DAQmxBase Create Task.vi"() -> ("task out"=w403:refnum<k21>, "error out"=w402:errorcluster)  [unwired: 14 in]
        n151 = call-poly <vilib>:"DAQmxBase Create Virtual Channel.vi"("task in"=w403, "physical channels"=tag "Dev1/ai0,Dev1/ai1,Dev1/ai2,Dev1/ai3", "error in"=w402) -> ("task out"=w400:refnum<k21>, "error out"=w401:errorcluster)  [unwired: 11 in]
        n152 = call-poly <vilib>:"DAQmxBase Timing.vi"("task/channels in"=w400, "sample mode"=w388, "rate"="Sample Rate", "error in"=w401) -> ("task out"=w399:refnum<k21>, "error out"=w398:errorcluster)  [unwired: 10 in]
        n153 = call "Functional Global I32.vi"("Enum"=enum16{"Set Data", "Get Data"}."Set Data", "Integer In"="Sample Rate") -> ()  [unwired: 9 in, 1 out]
        n154 = call <vilib>:"DAQmxBase Start Task.vi"("task/channels in"=w399, "error in"=w398) -> ("task out"=w397:refnum<k21>, "error out"=w387:errorcluster)  [unwired: 12 in]
        n155 = call <vilib>:"Simple Error Handler.vi"("error in (no error)"=w387) -> ()  [unwired: 4 in, 5 out]
      }
      frame "Exit" {
      }
    }
    n156 = Get Notifier Status(notifier=w341, error in (no error)=w340) -> (current notification=w342:bool)  [unwired: 4 out]
    n157 = Or(x=w352, y=w342) -> (x .or. y?=w343:bool)
  }
  n158 = Release Queue(queue=w27, error in (no error)=w26) -> ()  [unwired: 1 in, 3 out]
  n159 = Release Queue(queue=w25, error in (no error)=w24) -> (error out=w16:errorcluster)  [unwired: 1 in, 2 out]
  n160 = call <vilib>:"DAQmxBase Clear Task.vi"("task in"=w18, "error in"=w17) -> ("error out"=w15:errorcluster)  [unwired: 13 in]
  n161 = Merge Errors(w16, w15) -> (w14:errorcluster)
  n162 = call <vilib>:"Simple Error Handler.vi"("error in (no error)"=w14) -> ()  [unwired: 4 in, 5 out]
